vi "GetRTPCFlowPressure.vi"(0 "RTPC ID Number":i32) -> (1 "Flow":dbl, 2 "Pressure":dbl)   [LabVIEW 2011]
uses:
  GlobalVariables.vi
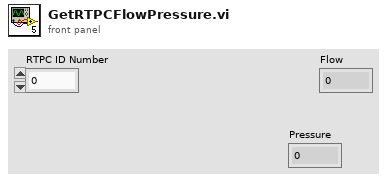
[diagram p1: front panel]
types:
  T1 = typedef "RTPC Cluster.ctl" = cluster{"ID Number":u8, "Status":bool[], "Flow (SCCM)":dbl, "Pressure (SCCM)":dbl, "Valve":i16, "Active Instance":i8, "Output":dbl}
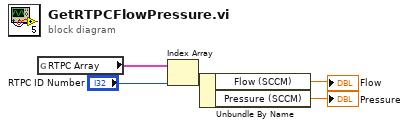
[diagram p0: block diagram]
diagram:
  n1 = global read "GlobalVariables.vi" "RTPC Array"() -> (w5:T1[])
  n2 = Index Array(array=w5, index="RTPC ID Number") -> (element=w4:T1)
  n3 = Unbundle By Name(w4) -> ("Flow (SCCM)"=→"Flow":dbl, "Pressure (SCCM)"=→"Pressure":dbl)
